vi "RegisterRead.vi"(6 "Compare Bits In":T1[](array[typedef]) {"Expected Value(s)" format="%.0x"}, 7 "Register Read/Write":T2 {"Register" format="%.0x"; "Slave Address" max=15 format="%.0x"}, 8 "error in (no error)":errorcluster, 9 "Number of Samples In":i32, 10 "Data Array":u8[][](array[numeric]), 11 "RFFE_Data In":T3 {"Toggle (high to low)" items=["0", "1", "Z", "L", "H", "X", "T", "V"]; "X Array" items=["0", "1", "Z", "L", "H", "X", "T", "V"]; "Z Array" items=["0", "1", "Z", "L", "H", "X", "T", "V"]; "L Array" items=["0", "1", "Z", "L", "H", "X", "T", "V"]; "H Array" items=["0", "1", "Z", "L", "H", "X", "T", "V"]; "One Array" items=["0", "1", "Z", "L", "H", "X", "T", "V"]; "Zero Array" items=["0", "1", "Z", "L", "H", "X", "T", "V"]}) -> (0 "error out":errorcluster, 1 "Number of Samples Out out":i32, 2 "Data Array Out":u8[][](array[numeric]), 3 "RFFE_Data Out":T3 {"Toggle (high to low)" items=["0", "1", "Z", "L", "H", "X", "T", "V"]; "X Array" items=["0", "1", "Z", "L", "H", "X", "T", "V"]; "Z Array" items=["0", "1", "Z", "L", "H", "X", "T", "V"]; "L Array" items=["0", "1", "Z", "L", "H", "X", "T", "V"]; "H Array" items=["0", "1", "Z", "L", "H", "X", "T", "V"]; "One Array" items=["0", "1", "Z", "L", "H", "X", "T", "V"]; "Zero Array" items=["0", "1", "Z", "L", "H", "X", "T", "V"]}, 4 "Compare Bits Out":T1[](array[typedef]) {"Expected Value(s)" format="%.0x"})   [LabVIEW 2013]
doc: "Builds MIPI RFFE Register Read with the specified data."
uses:
  Ctrls/RFFE_Data.ctl
  Ctrls/ClockDataChannels.ctl
  Ctrls/RegReadWrite.ctl
  Ctrls/ReadInfo.ctl
  Ctrls/Commands.ctl
  Ctrls/Read_Write_Data.ctl
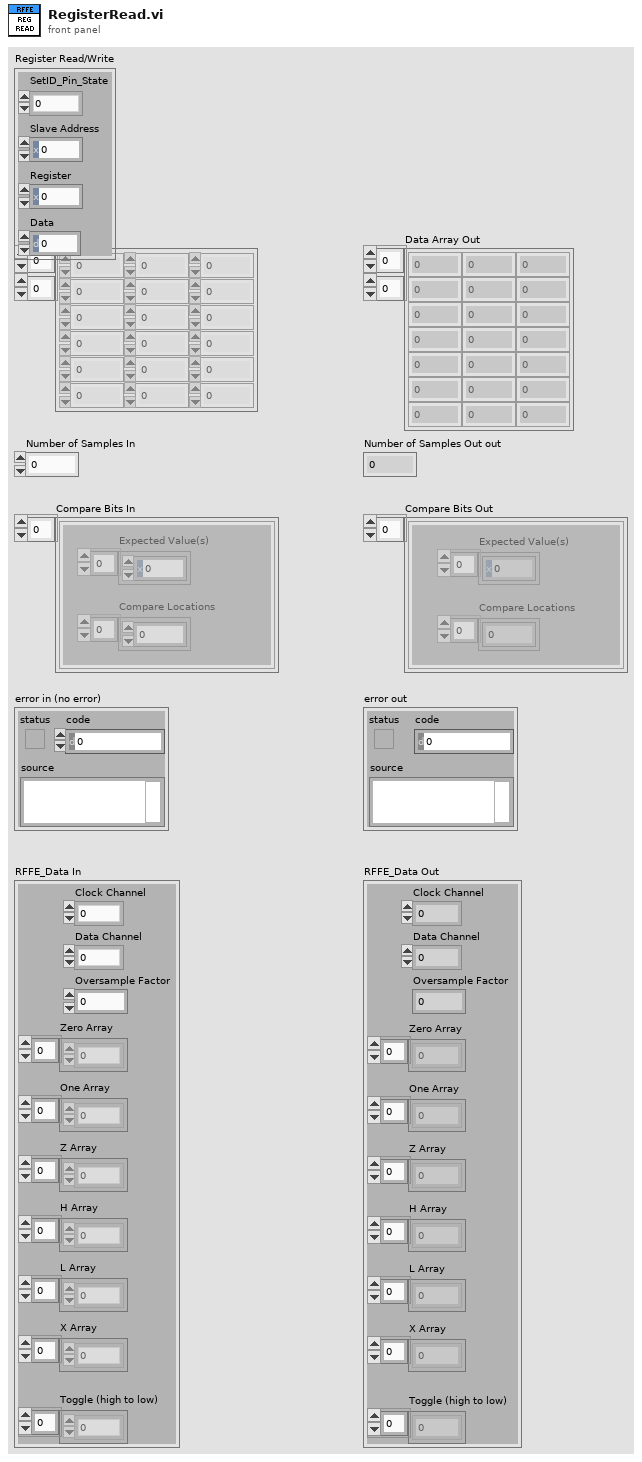
[diagram p1: front panel]
types:
  T1 = typedef "ReadInfo.ctl" = cluster{"Expected Value(s)":u8[], "Compare Locations":u32[]}
  T2 = typedef "RegReadWrite.ctl" = cluster{"Slave Address":u8, "Register":u8, "Data":u8, "SetID_Pin_State":enum16{"0", "1", "Z"}}
  T3 = typedef "RFFE_Data.ctl" = cluster{"Clock Channel":T4, "Data Channel":T4, "Oversample Factor":u8, "Zero Array":u8[], "One Array":u8[], "Z Array ":u8[], "H Array":u8[], "L Array":u8[], "X Array":u8[], "Toggle (high to low)":u8[]}
  T4 = typedef "ClockDataChannels.ctl" = enum16{"0", "1"}
  T5 = typedef "Read_Write_Data.ctl" = cluster{"Data":u8, "Read/Write":enum16{"Read", "Write"}}
  T6 = typedef "Commands.ctl" = cluster{"Command":enum16{"Extended Register Write", "Extended Register Read", "Extended Register Write Long", "Extended Register Read Long", "Register Write", "Register Read", "Register 0 Write"}, "Data/Address/ByteCount":u8}
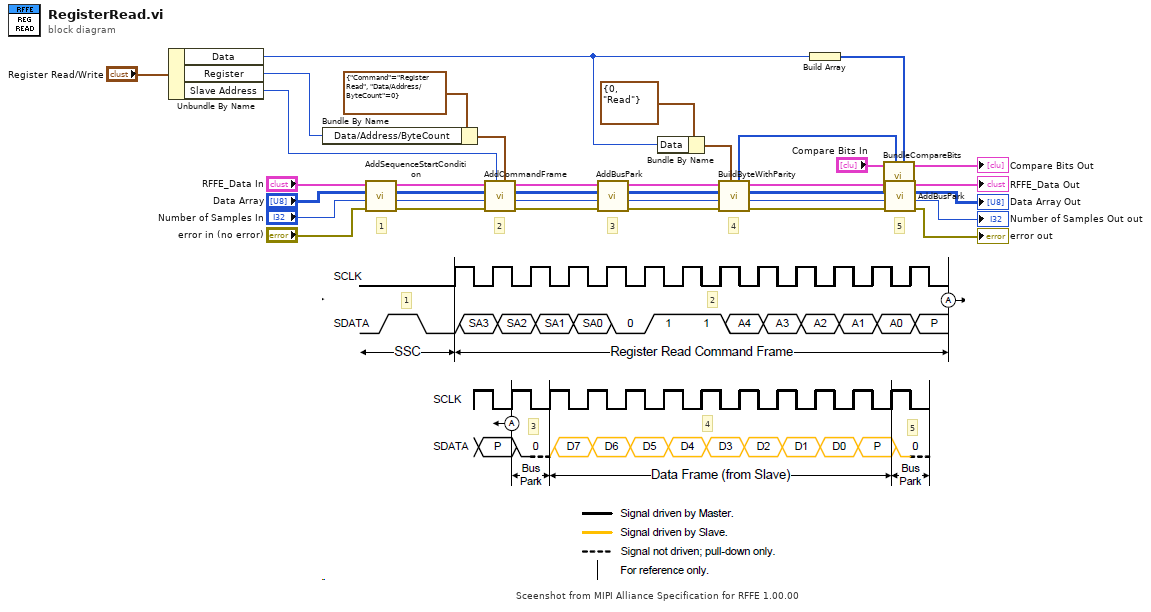
[diagram p0: block diagram]
diagram:
  # "Sceenshot from MIPI Alliance Specification for RFFE 1.00.00"
  # "5"
  # "4"
  # "3"
  # "2"
  # "1"
  # "5"
  # "4"
  # "3"
  # "2"
  # "1"
  n1 = Unbundle By Name("Register Read/Write") -> ("Data"=w5:u8, "Register"=w21:u8, "Slave Address"=w12:u8)
  n2 = Bundle By Name(cluster=T6 {"Command"=enum."Register Read", "Data/Address/ByteCount"=0} ("Command"), "Data/Address/ByteCount"=w21) -> (w13:T6)
  n3 = call "AddSequenceStartCondition.vi"("error in (no error)"="error in (no error)", "Number of Samples In"="Number of Samples In", "Data Array In"="Data Array", "RFFE_Data In"="RFFE_Data In") -> ("error out"=w31:errorcluster, "Number of Samples Out"=w34:i32, "Data Array Out"=w32:u8[][], "RFFE_Data Out"=w33:T3)  [unwired: 4 in]
  n4 = call "AddCommandFrame.vi"("Command"=w13, "Slave Address"=w12, "error in (no error)"=w31, "Number of Samples In"=w34, "Data Array In"=w32, "RFFE_Data"=w33) -> ("error out"=w18:errorcluster, "Number of Samples Out"=w17:i32, "Data Array Out"=w16:u8[][], "Configuratation Out"=w19:T3)  [unwired: 2 in]
  n5 = call "AddBusPark.vi"("error in (no error)"=w18, "Number of Samples In"=w17, "Data Array In"=w16, "RFFE_Data In"=w19) -> ("error out"=w10:errorcluster, "Number of Samples Out"=w7:i32, "Data Array Out"=w8:u8[][], "RFFE_Data Out"=w9:T3)  [unwired: 4 in]
  n6 = Bundle By Name(cluster=T5 {"Data"=0, "Read/Write"=enum."Read"} ("Read/Write Data"), "Data"=w5) -> (w20:T5)
  n7 = call "BuildByteWithParity.vi"("Read/Write Data"=w20, "error in"=w10, "Number of Samples In"=w7, "Data Array In"=w8, "RFFE_Data In"=w9) -> ("error out"=w15:errorcluster, "Number of Samples Out"=w23:i32, "Data Array Out"=w24:u8[][], "RFFE_Data Out"=w3:T3, "Compare Locations"=w6:u32[])  [unwired: 2 in]
  n8 = Build Array(w5) -> (w4:u8[])
  n9 = call "BundleCompareBits.vi"("Expected Value(s)"=w4, "Compare Locations"=w6, "Compare Bits In"="Compare Bits In") -> ("Compare Bits Out"=→"Compare Bits Out":T1[])  [unwired: 8 in]
  n10 = call "AddBusPark.vi"("error in (no error)"=w15, "Number of Samples In"=w23, "Data Array In"=w24, "RFFE_Data In"=w3) -> ("error out"=→"error out":errorcluster, "Number of Samples Out"=→"Number of Samples Out out":i32, "Data Array Out"=→"Data Array Out":u8[][], "RFFE_Data Out"=→"RFFE_Data Out":T3)  [unwired: 4 in]
